vi "Lab_2_Framework.vi"() -> ()   [LabVIEW 2025]
uses:
  <vilib>/Analysis/3filter.llb/Filter Passband Type.ctl
  LVLib/SADI_FW3.lvlib
  <vilib>/ptbypt/NI_PtbyPt.lvlib
  <vilib>/Analysis/NI_AALBase.lvlib
panel:
  in  "pid/bb":bool
  in  "Kd":dbl
  in  "Ki":dbl
  in  "Kp":dbl
  out "error":dbl
  in  "Couts/rev":dbl=3704.0
  in  "Tab Control":T1(tab)=enum."Stuff you need to use"
  in  "Latest?":bool=TRUE
  out "SADIs Connected":u32=1
  in  "instance":i32
  in  "Loop Frequency":u16=30000 min=1
  out "MSG CNT":u32=403028
  in  "Mode Select":T2(ring)=enum."daqMode_pendulum"
  in  "Encoder Pin Location 1":u16(ring)=2 items=["D0"=0, "D1"=1, "D2"=2, "D3"=3, "D4"=4, "D5"=5, "D6"=6, "D8"=8, "D9"=9, "D10"=10, "D11"=11]
  in  "Encoder Pin Location 0":u16(ring) items=["D0"=0, "D1"=1, "D2"=2, "D3"=3, "D4"=4, "D5"=5, "D6"=6, "D8"=8, "D9"=9, "D10"=10, "D11"=11]
  in  "OutputPinMsk":u16=240 format="%x"
  in  "servoEnableMask":u8 format="%x"
  in  "motorEnableMask":u8 format="%x"
  out "Setup Valid":bool=TRUE
  out "Stopped":bool=TRUE
  in  "Output Units":enum16{"Degrees", "Radians"}(ring)
  out "PendEncValMax":u16=500
  in  "ADC GAIN 0":u16(ring)=2 items=["Range_CH_OFF_msk"=0, "Range_pm_10_24_msk"=1, "Range_pm_05_12_msk"=2, "Range_pm_02_56_msk"=3, "Range_pm_01_28_msk"=4, "Range_pm_00_64_msk"=5, "Range_10_24_msk"=9, "Range_05_12_msk"=10, "Range_02_56_msk"=11, "Range_01_28_msk"=12]
  in  "ADC GAIN 3":u16(ring)=2 items=["Range_CH_OFF_msk"=0, "Range_pm_10_24_msk"=1, "Range_pm_05_12_msk"=2, "Range_pm_02_56_msk"=3, "Range_pm_01_28_msk"=4, "Range_pm_00_64_msk"=5, "Range_10_24_msk"=9, "Range_05_12_msk"=10, "Range_02_56_msk"=11, "Range_01_28_msk"=12]
  in  "ADC GAIN 2":u16(ring)=2 items=["Range_CH_OFF_msk"=0, "Range_pm_10_24_msk"=1, "Range_pm_05_12_msk"=2, "Range_pm_02_56_msk"=3, "Range_pm_01_28_msk"=4, "Range_pm_00_64_msk"=5, "Range_10_24_msk"=9, "Range_05_12_msk"=10, "Range_02_56_msk"=11, "Range_01_28_msk"=12]
  in  "ADC GAIN 1":u16(ring)=2 items=["Range_CH_OFF_msk"=0, "Range_pm_10_24_msk"=1, "Range_pm_05_12_msk"=2, "Range_pm_02_56_msk"=3, "Range_pm_01_28_msk"=4, "Range_pm_00_64_msk"=5, "Range_10_24_msk"=9, "Range_05_12_msk"=10, "Range_02_56_msk"=11, "Range_01_28_msk"=12]
  out "FT_ERROR_ENUM":T3(ring)=enum."FT_INVALID_HANDLE"
  out "Loop Time (ms)":dbl=0.241100000039296 format="%.6f"
  in  "Encoder Resolution 0":u16=360
  in  "Encoder Resolution 1":u16=360
  out "PendEncValMin":u16=10000
  out "Software Version":dbl=3.024 format="%_6g"
  out "Firmware Version":sgl=3.41
  out "Motor Rotation Counts":i32=1147
  out "Motor Velocity":i32=64951
  in  "Cutoff freq: fl":dbl=40.0 format="%0.3f"
  in  "Sampling freq: fs":dbl=2000.0
  in  "initialize":bool
  out "Filtered Platen Rotation Angle":dbl format="%0.2f"
  out "Platen Velocity":dbl
  out "Total Angle":dbl
  in  "Zero":bool
  in  "Amplitude":dbl=300.0
  in  "Turn On Command":dbl=90.0
  in  "Frequency":dbl=0.5
  in  "Sine (L)/Square (R)":bool
  in  "Enable Motor":bool=TRUE
  in  "Stop":bool=TRUE
  in  "Desired Loop \nTime (ms)":dbl=0.5
  out "Actual Loop \nTime (ms)":dbl
  out "Elapsed \nTime (s)":dbl
  out "Segments Saved":u32
  in  "Save Data?":bool
  out "Platen Rotation Graph":dbl[](graph)=[-15.548225345013767, -16.52267818574514]
  out "Platen Vel Graph":dbl[](graph)=[-331.020601457828, -300.0]
  out "Command Signal Graph":dbl[](graph)=[-300.0]
  out "Command Signal":dbl
  in  "d":dbl
  in  "duty cycle":dbl
  in  "Reset mt":bool
  in  "n-int":i32 caption="n int"
  in  "n-diff":i32 caption="n diff"
  out "Read Call Error Out":u16(ring)=32768 items=["SADI_RESET (FT_OK)"=0, "FT_INVALID_HANDLE"=1, "FT_DEVICE_NOT_FOUND"=2, "FT_DEVICE_NOT_OPENED"=3, "FT_IO_ERROR"=4, "FT_INSUFFICIENT_RESOURCES"=5, "FT_OTHER_ERROR"=18, "FT_NOT_SUPPORTED"=17, "DATA_RECEIVED"=32768, "NO_DATA_AVAIL"=32769, "NO_SADI"=32770]
  out "SADI State":T4(ring)=enum."Run_state"
  # "Platen Rotation & Velocity"
  # "Signal Generator"
  # "Butterworth Filter Settings"
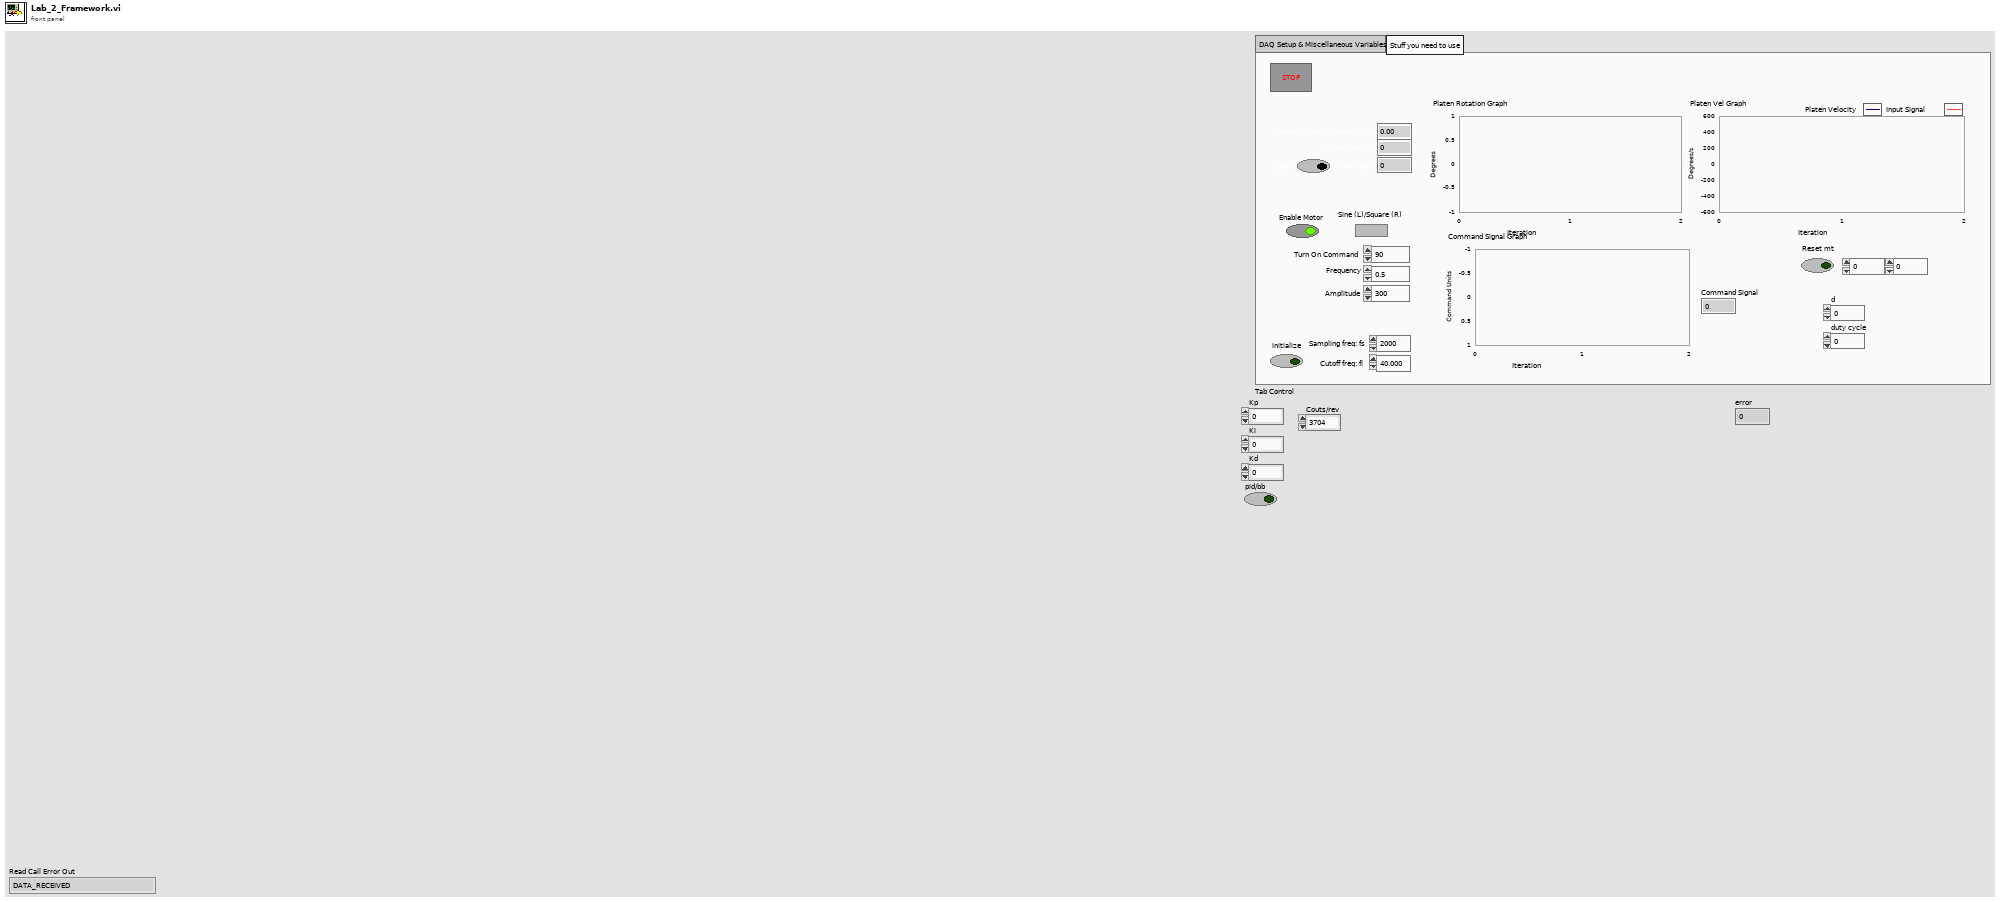
[diagram p1: front panel]
types:
  T1 = enum32{"DAQ Setup & Miscellaneous Variables", "Stuff you need to use"}
  T2 = enum16{"daqMode_unassigned", "daqMode_generic", "daqMode_pendulum", "daqMode_mom"}
  T3 = enum32{"FT_OK", "FT_INVALID_HANDLE", "FT_DEVICE_NOT_FOUND", "FT_DEVICE_NOT_OPENED", "FT_IO_ERROR", "FT_INSUFFICIENT_RESOURCES", "FT_INVALID_PARAMETER", "FT_INVALID_BAUD_RATE", "FT_DEVICE_NOT_OPENED_FOR_ERASE", "FT_DEVICE_NOT_OPENED_FOR_WRITE", "FT_FAILED_TO_WRITE_DEVICE", "FT_EEPROM_READ_FAILED", "FT_EEPROM_WRITE_FAILED", "FT_EEPROM_ERASE_FAILED", "FT_EEPROM_NOT_PRESENT", "FT_EEPROM_NOT_PROGRAMMED", "FT_INVALID_ARGS", "FT_NOT_SUPPORTED", "FT_OTHER_ERROR", "FT_DEVICE_LIST_NOT_READY"}
  T4 = enum32{"NotOpened_state", "Opened_state", "Ready_state", "Setup_state", "InitSent_state", "Start_initiated_state", "Run_state", "StopInitiated_state", "Stopped_state"}
  T5 = typedef "NI_AALBase.lvlib/Filter Passband Type.ctl" = enum32{"Lowpass", "Highpass", "Bandpass", "Bandstop"}
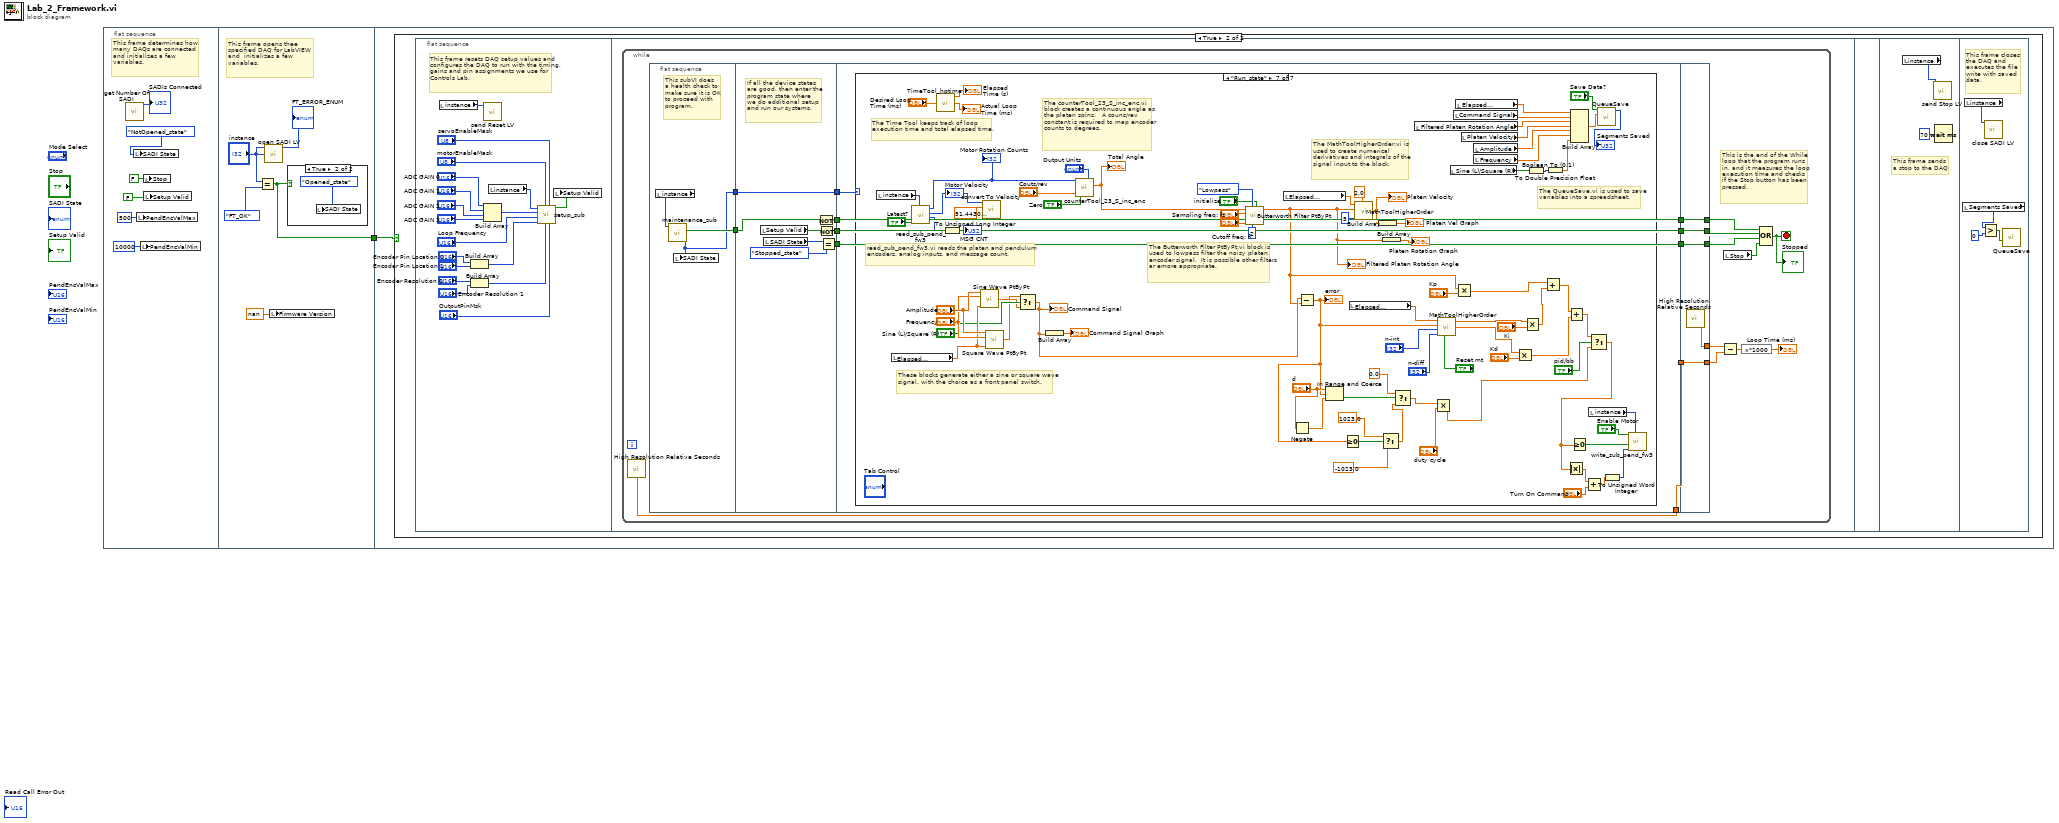
[diagram p0: block diagram]
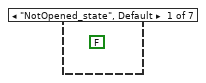
[diagram p4: hidden frame]
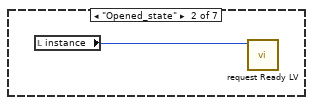
[diagram p5: hidden frame]
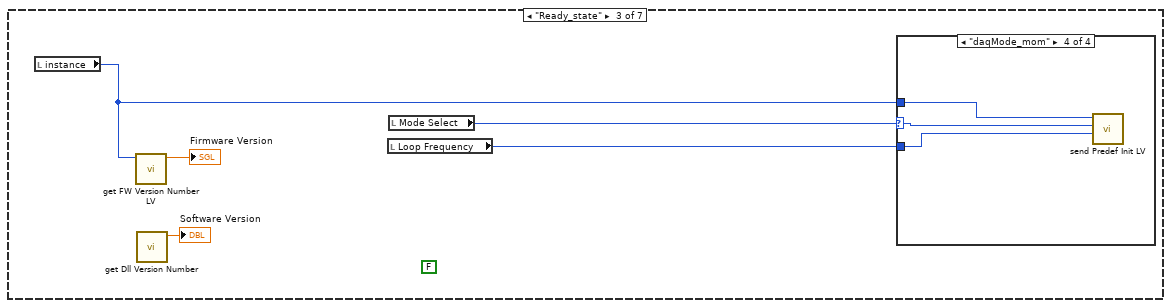
[diagram p6: hidden frame]
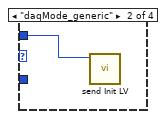
[diagram p8: hidden frame]
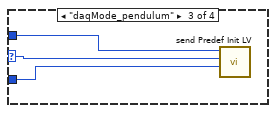
[diagram p9: hidden frame]
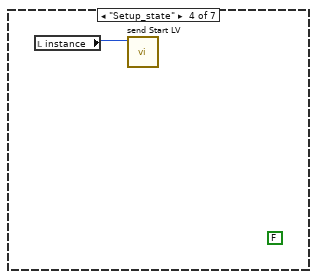
[diagram p10: hidden frame]
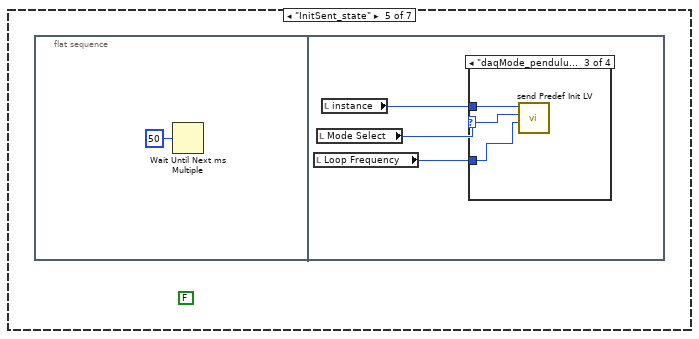
[diagram p11: hidden frame]
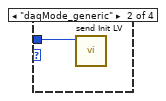
[diagram p13: hidden frame]
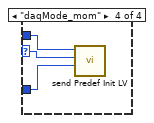
[diagram p14: hidden frame]
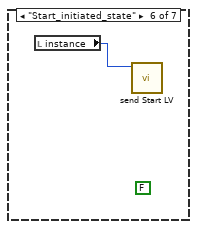
[diagram p15: hidden frame]
diagram:
  n1 = flat-sequence {
    tunnel: [w10] -> w1
    tunnel: w1 -> [w14]
    frame #0 {
      # "This frame determines how many DAQs are connected and initializes a few variables."
      n2 = call "get Number Of SADI.vi"() -> ("function return"=→"SADIs Connected":u32)  [unwired: 11 in]
      n3 = local write "SADI State"(T4."NotOpened_state" ("SADI State")) -> ()
      n4 = local write "PendEncValMax"(u16 500 ("PendEncValMax")) -> ()
      n5 = local write "PendEncValMin"(u16 10000 ("PendEncValMin")) -> ()
      n6 = local write "Stop"(FALSE ("Stop")) -> ()
      n7 = local write "Setup Valid"(FALSE ("Setup Valid")) -> ()
    }
    frame #1 {
      # "This frame opens thee specified DAQ for LabVIEW and  initializes a few variables."
      n8 = Equal?(x="instance", y=T3."FT_OK" ("FT_ERROR_ENUM 2")) -> (x = y?=w10:bool)
      n9 = call "open SADI LV.vi"("deviceNumber"="instance", "instance"="instance") -> ("function return"=→"FT_ERROR_ENUM":u32)  [unwired: 9 in]
      n10 = local write "Firmware Version"(nan ("Firmware Version")) -> ()
      n11 = case shown="True" w10 {
        frame False {
        }
        frame True {
          n12 = local write "SADI State"(T4."Opened_state" ("SADI State 2")) -> ()
        }
      }
    }
    frame #2 {
      n13 = case shown="True" w14 {
        frame False {
        }
        frame True {
          n14 = flat-sequence {
            frame #0 {
              # "This frame resets DAQ setup values and configures the DAQ to run with the timing, gains and pin assignments we use for Controls Lab."
              n15 = local read "instance"() -> (w16:i32)
              n16 = Build Array("Encoder Pin Location 0", "Encoder Pin Location 1") -> (w26:u16[])
              n17 = Build Array("Encoder Resolution 0", "Encoder Resolution 1") -> (w23:u16[])
              n18 = Build Array("ADC GAIN 0", "ADC GAIN 1", "ADC GAIN 2", "ADC GAIN 3") -> (w28:u16[])
              n19 = call "send Reset LV.vi"("instance"=w16) -> ()  [unwired: 11 in]
              n20 = local read "instance"() -> (w17:i32)
              n21 = call "setup_sub.vi"("OutputPinMsk"="OutputPinMsk", "servoEnableMask"="servoEnableMask", "ENC_RES_Array"=w23, "motorEnableMask"="motorEnableMask", "pinLocation_Array"=w26, "Loop Frequency"="Loop Frequency", "ADC_Settings"=w28, "instance"=w17) -> ("Success?"=w18:bool)  [unwired: 3 in]
              n22 = local write "Setup Valid"(w18) -> ()
            }
            frame #1 {
              n23 = while {
                stop <- w47 stop-if-true
                # "This is the end of the While \nloop that the program runs\nin, and it measures the loop\nexecution time and checks\nif the Stop button has been\npressed."
                n24 = call <vilib>:"High Resolution Relative Seconds.vi"() -> ("relative seconds"=w35:dbl)
                n25 = flat-sequence {
                  tunnel: [w55] -> w52
                  tunnel: [w53] -> w33
                  tunnel: w52 -> [w60]
                  tunnel: [w59] -> w46
                  tunnel: [w58] -> w45
                  tunnel: [w57] -> w44
                  tunnel: [w56] -> w34
                  tunnel: w33 -> [w56]
                  tunnel: w46 -> [w68]
                  tunnel: w45 -> [w67]
                  tunnel: w44 -> [w66]
                  tunnel: [w68] -> w43
                  tunnel: [w67] -> w42
                  tunnel: [w66] -> w41
                  tunnel: [w65] -> w39
                  tunnel: w35 -> [w65]
                  tunnel: w34 -> [w64]
                  tunnel: [w178] -> w49
                  tunnel: [w179] -> w50
                  tunnel: [w180] -> w51
                  tunnel: w43 -> [w180]
                  tunnel: w42 -> [w179]
                  tunnel: w41 -> [w178]
                  tunnel: [w177] -> w40
                  tunnel: w39 -> [w176]
                  tunnel: [w176] -> w38
                  frame #0 {
                    # "This subVI does\na health check to\nmake sure it is OK\nto proceed with\nprogram."
                    n26 = local read "instance"() -> (w54:i32)
                    n27 = call "maintenance_sub.vi"("Instance"=w54) -> ("SADI State"=w53:T4, "FT_OK?"=w55:bool)  [unwired: 8 in, 1 out]
                    n28 = local write "SADI State"(w53) -> ()
                  }
                  frame #1 {
                    # "If all the device states\nare good, then enter the\nprogram state where\nwe do additional setup\nand run our systems."
                    n29 = local read "Setup Valid"() -> (w63:bool)
                    n30 = local read "SADI State"() -> (w61:T4)
                    n31 = Not(x=w60) -> (.not. x?=w59:bool)
                    n32 = Not(x=w63) -> (.not. x?=w58:bool)
                    n33 = Equal?(x=w61, y=T4."Stopped_state") -> (x = y?=w57:bool)
                  }
                  frame #2 {
                    n34 = case shown="\"Run_state\"" w64 {
                      frame "NotOpened_state", Default {
                        (unwired) FALSE ("dataToRead?")
                      }
                      frame "Opened_state" {
                        n35 = local read "instance"() -> (w69:i32)
                        n36 = call "request Ready LV.vi"("instance"=w69) -> ()  [unwired: 11 in]
                      }
                      frame "Ready_state" {
                        (unwired) FALSE ("dataToRead?")
                        n37 = local read "instance"() -> (w72:i32)
                        n38 = call "get FW Version Number LV.vi"("instance"=w72) -> ("function return"=→"Firmware Version":dbl)  [unwired: 10 in]
                        n39 = call "get Dll Version Number.vi"() -> ("function return"=→"Software Version":dbl)  [unwired: 11 in]
                        n40 = local read "Loop Frequency"() -> (w70:u16)
                        n41 = local read "Mode Select"() -> (w71:T2)
                        n42 = case shown="\"daqMode_mom\"" w71 {
                          selector: w71 -> [_ _ w77 w80]
                          tunnel: w72 -> [_ w75 w78 w81]
                          tunnel: w70 -> [_ _ w76 w79]
                          frame "daqMode_unassigned", Default {
                          }
                          frame "daqMode_generic" {
                            n43 = call "send Init LV.vi"("instance"=w75) -> ()  [unwired: 11 in]
                          }
                          frame "daqMode_pendulum" {
                            n44 = call "send Predef Init LV.vi"("freq"=w76, "selection"=w77, "instance"=w78) -> ()  [unwired: 9 in]
                          }
                          frame "daqMode_mom" {
                            n45 = call "send Predef Init LV.vi"("freq"=w79, "selection"=w80, "instance"=w81) -> ()  [unwired: 9 in]
                          }
                        }
                      }
                      frame "Setup_state" {
                        (unwired) FALSE ("dataToRead?")
                        n46 = local read "instance"() -> (w82:i32)
                        n47 = call "send Start LV.vi"("instance"=w82) -> ()  [unwired: 11 in]
                      }
                      frame "InitSent_state" {
                        (unwired) FALSE ("dataToRead?")
                        n48 = flat-sequence {
                          frame #0 {
                            n49 = Wait Until Next ms Multiple(millisecond multiple=u32 50) -> ()  [unwired: 1 out]
                          }
                          frame #1 {
                            n50 = local read "Loop Frequency"() -> (w84:u16)
                            n51 = local read "Mode Select"() -> (w85:T2)
                            n52 = local read "instance"() -> (w86:i32)
                            n53 = case shown="\"daqMode_pendulum\"" w85 {
                              selector: w85 -> [_ _ w90 w92]
                              tunnel: w86 -> [_ w87 w89 w93]
                              tunnel: w84 -> [_ _ w88 w91]
                              frame "daqMode_unassigned", Default {
                              }
                              frame "daqMode_generic" {
                                n54 = call "send Init LV.vi"("instance"=w87) -> ()  [unwired: 11 in]
                              }
                              frame "daqMode_pendulum" {
                                n55 = call "send Predef Init LV.vi"("freq"=w88, "selection"=w90, "instance"=w89) -> ()  [unwired: 9 in]
                              }
                              frame "daqMode_mom" {
                                n56 = call "send Predef Init LV.vi"("freq"=w91, "selection"=w92, "instance"=w93) -> ()  [unwired: 9 in]
                              }
                            }
                          }
                        }
                      }
                      frame "Start_initiated_state" {
                        (unwired) FALSE ("dataToRead?")
                        n57 = local read "instance"() -> (w94:i32)
                        n58 = call "send Start LV.vi"("instance"=w94) -> ()  [unwired: 11 in]
                      }
                      frame "Run_state" {
                        # "The counterTool_23_S_inc_enc.vi block creates a continuous angle as the platen spins.   A couns/rev constant is required to map encoder counts to degrees."
                        # "The QueueSave.vi is used to save variables into a spreadsheet."
                        # "The MathToolHigherOrder.vi is used to create numerical derivatives and integrals of the signal input to the block."
                        # "The Butterworth Filter PtByPt.vi block is used to lowpass filter the noisy platen encoder signal.  It is possible other filters ar emore appropriate."
                        # "These blocks generate either a sine or square wave signal, with the choice as a front panel switch."
                        # "read_sub_pend_fw3.vi reads the platen and pendulum encoders, analog inputs, and message count."
                        # "The Time Tool keeps track of loop execution time and total elapsed time."
                        n59 = local read "instance"() -> (w173:i32)
                        n60 = local read "Elapsed \nTime (s)"() -> (w129:dbl)
                        n61 = call "read_sub_pend_fw3.vi"("instance"=w173, "Latest?"="Latest?") -> ("MSG CNT"=w171:u32, "ENC VEL 0"=w138:u16, "ENC POS 0"=w125:i32)  [unwired: 6 in, 1 out]
                        "Motor Velocity" <- w138
                        "Motor Rotation Counts" <- w125
                        n62 = call "TimeTool_hptime.vi"("Desired Loop Time (ms)"="Desired Loop \nTime (ms)") -> ("elapsed time (s)"=→"Elapsed \nTime (s)":dbl, "dt (ms)"=→"Actual Loop \nTime (ms)":dbl)  [unwired: 1 out]
                        n63 = To Unsigned Long Integer(number=w171) -> (unsigned 32bit integer=→"MSG CNT":u32)
                        n64 = call <vilib>:"Sine Wave PtByPt.vi"("time"=w129, "frequency"="Frequency", "amplitude"="Amplitude") -> ("sine wave"=w127:dbl)  [unwired: 1 in]
                        n65 = call "convert To Velocity.vi"("gearRatio"=sgl 51.443, "velVal"=w138) -> ()  [unwired: 9 in, 1 out]
                        n66 = call <vilib>:"Square Wave PtByPt.vi"("amplitude"="Amplitude", "frequency"="Frequency", "time"=w129) -> ("square wave"=w126:dbl)  [unwired: 2 in]
                        n67 = Select(t=w126, s="Sine (L)/Square (R)", f=w127) -> (s? t:f=w124:dbl)
                        "Command Signal" <- w124
                        n68 = Build Array(w124) -> (→"Command Signal Graph":dbl[])
                        n69 = call "counterTool_23_S_inc_enc.vi"("Counts"=w125, "Zero"="Zero", "Couts/rev"="Couts/rev", "Output Units"="Output Units") -> ("Total Angle"=w139:dbl)  [unwired: 3 in, 1 out]
                        "Total Angle" <- w139
                        n70 = call <vilib>:"Butterworth Filter PtByPt.vi"("initialize"="initialize", "order"=2, "filter type"=Filter_Passband_Type."Lowpass", "low cutoff freq: fl"="Cutoff freq: fl", "sampling freq: fs"="Sampling freq: fs", "x"=w139) -> ("Filtered x"=w108:dbl)  [unwired: 3 in, 1 out]
                        "Filtered Platen Rotation Angle" <- w108
                        n71 = local read "Elapsed \nTime (s)"() -> (w162:dbl)
                        n72 = Negate(x="d") -> (-x=w122:dbl)
                        n73 = Subtract(x=w124, y=w108) -> (x-y=w112:dbl)
                        "error" <- w112
                        n74 = In Range and Coerce(upper limit="d", x=w112, lower limit=w122) -> (In Range?=w120:bool)  [unwired: 1 out]
                        n75 = Greater Or Equal To 0?(x=w112) -> (x >= 0?=w119:bool)
                        n76 = local read "Elapsed \nTime (s)"() -> (w113:dbl)
                        n77 = call "MathToolHigherOrder.vi"("Time"=w162, "Interp Order (NaN for Npts-1)"=2.0, "Data"=w108, "n-diff"=5) -> ("1st derivative"=w141:dbl)  [unwired: 2 in, 2 out]
                        "Platen Velocity" <- w141
                        n78 = Build Array(w141) -> (→"Platen Vel Graph":dbl[])
                        n79 = Select(t=1023.0, s=w119, f=-1023.0) -> (s? t:f=w116:dbl)
                        n80 = Build Array(w108) -> (→"Platen Rotation Graph":dbl[])
                        n81 = Select(t=0.0, s=w120, f=w116) -> (s? t:f=w115:dbl)
                        n82 = local read "Filtered Platen Rotation Angle"() -> (w150:dbl)
                        n83 = Multiply(x=w115, y="duty cycle") -> (x*y=w97:dbl)
                        n84 = call "MathToolHigherOrder.vi"("Time"=w113, "Data"=w112, "n-int"="n-int", "Reset (F)"="Reset mt", "n-diff"="n-diff") -> ("integral"=w105:dbl, "1st derivative"=w103:dbl)  [unwired: 1 in, 1 out]
                        n85 = local read "Sine (L)/Square (R)"() -> (w144:bool)
                        n86 = local read "Command Signal"() -> (w151:dbl)
                        n87 = Multiply(x=w108, y="Kp") -> (x*y=w102:dbl)
                        n88 = local read "Elapsed \nTime (s)"() -> (w166:dbl)
                        n89 = local read "Platen Velocity"() -> (w149:dbl)
                        n90 = local read "Amplitude"() -> (w147:dbl)
                        n91 = local read "Frequency"() -> (w146:dbl)
                        n92 = Multiply(x=w103, y="Kd") -> (x*y=w99:dbl)
                        n93 = Multiply(x=w105, y="Ki") -> (x*y=w101:dbl)
                        n94 = Boolean To (0,1)(Boolean=w144) -> (0, 1=w143:i16)
                        n95 = Add(x=w102, y=w101) -> (x+y=w100:dbl)
                        n96 = To Double Precision Float(number=w143) -> (double precision float=w145:dbl)
                        n97 = Add(x=w100, y=w99) -> (x+y=w98:dbl)
                        n98 = Build Array(w166, w151, w150, w149, w147, w146, w145) -> (w168:dbl[])
                        n99 = local read "instance"() -> (w148:i32)
                        n100 = Select(t=w98, s="pid/bb", f=w97) -> (s? t:f=w95:dbl)
                        n101 = Absolute Value(x=w95) -> (abs(x)=w136:dbl)
                        n102 = Greater Or Equal To 0?(x=w95) -> (x >= 0?=w154:bool)
                        n103 = Add(x=w136, y="Turn On Command") -> (x+y=w135:dbl)
                        n104 = call "QueueSave.vi"("Data In"=w168, "Save Data?"="Save Data?") -> ("Segments Saved"=→"Segments Saved":u32)  [unwired: 3 in, 2 out]
                        n105 = To Unsigned Word Integer(number=w135) -> (unsigned 16bit integer=w134:u16)
                        n106 = call "write_sub_pend_fw3.vi"("instance"=w148, "pendMotorVal"=w134, "pendDir"=w154, "enableWrite"="Enable Motor") -> ()  [unwired: 8 in]
                      }
                    }
                  }
                  frame #3 {
                    n107 = call <vilib>:"High Resolution Relative Seconds.vi"() -> ("relative seconds"=w177:dbl)
                  }
                }
                n108 = Subtract(x=w40, y=w38) -> (x-y=w37:dbl)
                n109 = local read "Stop"() -> (w48:bool)
                n110 = expression code="x*1000"(w37) -> (→"Loop Time (ms)":dbl)
                n111 = Compound Arithmetic op=OR(w51, w50, w49, w48) -> (w47:bool)
                "Stopped" <- w47
              }
            }
            frame #2 {
            }
            frame #3 {
              # "This frame sends\na stop to the DAQ"
              n112 = local read "instance"() -> (w182:i32)
              n113 = call "send Stop LV.vi"("instance"=w182) -> ()  [unwired: 11 in]
              n114 = Wait (ms)(milliseconds to wait=u32 70) -> ()  [unwired: 1 out]
            }
            frame #4 {
              # "This frame closes\nthe DAQ and \nexecutes the file\nwrite with saved\ndata."
              n115 = local read "Segments Saved"() -> (w185:u32)
              n116 = local read "instance"() -> (w186:i32)
              n117 = Greater?(x=w185, y=u32 0) -> (0:w184:bool)
              n118 = call "close SADI LV.vi"("instance"=w186) -> ()  [unwired: 10 in, 1 out]
              n119 = call "QueueSave.vi"("Write To Spreadsheet"=w184) -> ()  [unwired: 4 in, 3 out]
            }
          }
        }
      }
    }
  }
